vi "BioFeedback4(DAQ+ModularDesign).vi"() -> ()   [LabVIEW 2016]
uses:
  <vilib>/Analysis/5stat.llb/RMS (DBL).vi
  <vilib>/Analysis/NI_AALPro.lvlib
panel:
  out "initialized array size 2":dbl
  in  "Frames Per Second 2":dbl
  in  "Sample rate (Hz) 2":dbl=22050.0 caption="Sample rate (Hz)"
  out "Thermometer Elapsed Frames 2":i32
  out "(INTERNAL) Buffer Index 2":i32
  out "Moving Average num samples 2":i32
  out "AggregateSignalData 2":waveform(dbl)[](array[waveform])
  in  "Moving Average Length (s) 2":dbl
  out "rectified 4":waveform(dbl)[](graph)
  out "Data Levels 2":dbl(slide) scale=0.0..0.07
  out "rms data 2":dbl(graph)
  out "rectified 3":waveform(dbl)[](graph)
  out "raw input 2":waveform(dbl)(graph)
  out "aggregate signal 2":waveform(dbl)[](graph)
  out "initialized array size":dbl
  out "rectified 2":waveform(dbl)[](graph)
  out "number of resets":dbl
  in  "Frames Per Second":dbl
  in  "Sample rate (Hz)":dbl=22050.0
  out "Thermometer Elapsed Frames":i32
  out "(INTERNAL) Buffer Index":i32
  out "Moving Average num samples":i32
  out "AggregateSignalData":waveform(dbl)[](array[waveform])
  in  "Moving Average Length (s)":dbl
  out "rectified":waveform(dbl)[](graph)
  out "Data Levels":dbl(slide) scale=0.0..0.07
  out "rms data":dbl(graph)
  out "raw input":waveform(dbl)(graph)
  out "aggregate signal":waveform(dbl)[](graph)
  in  "Trial":dbl
  in  "Start":bool
  in  "Stop Recording":bool
  # "Biofeedback"
  # "Internal"
  # "Settings"
  # "Filter Settings"
  # "Bandpass Filter"
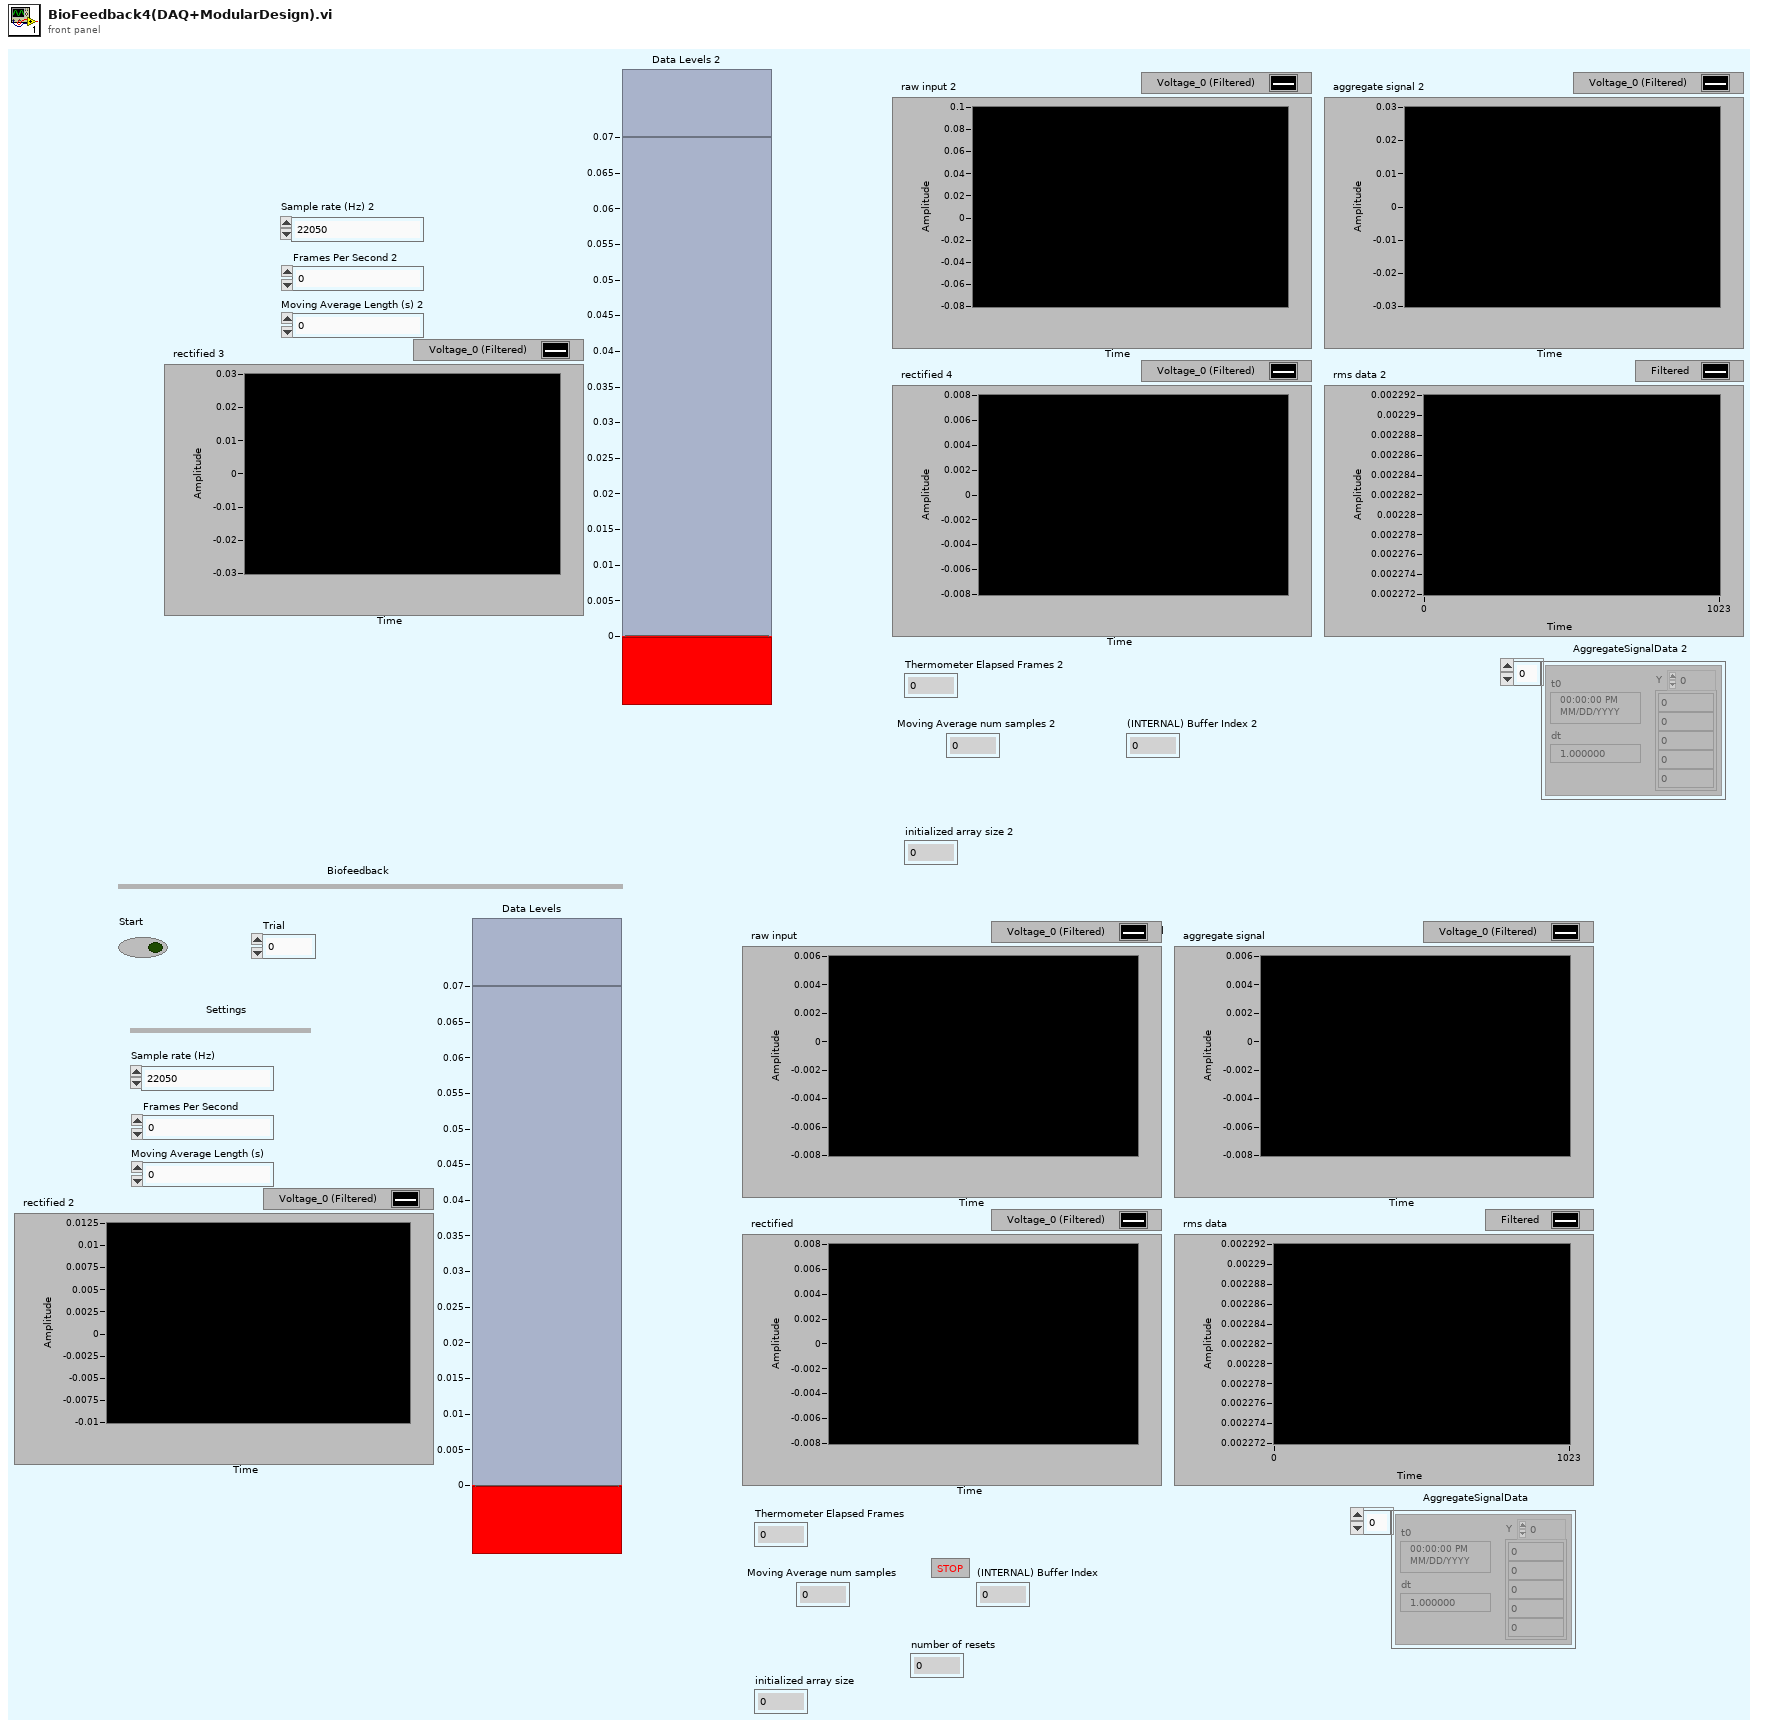
[diagram p1: front panel]
types:
  T1 = typedef "WaveformArrayControl.ctl" = waveform(dbl)[]
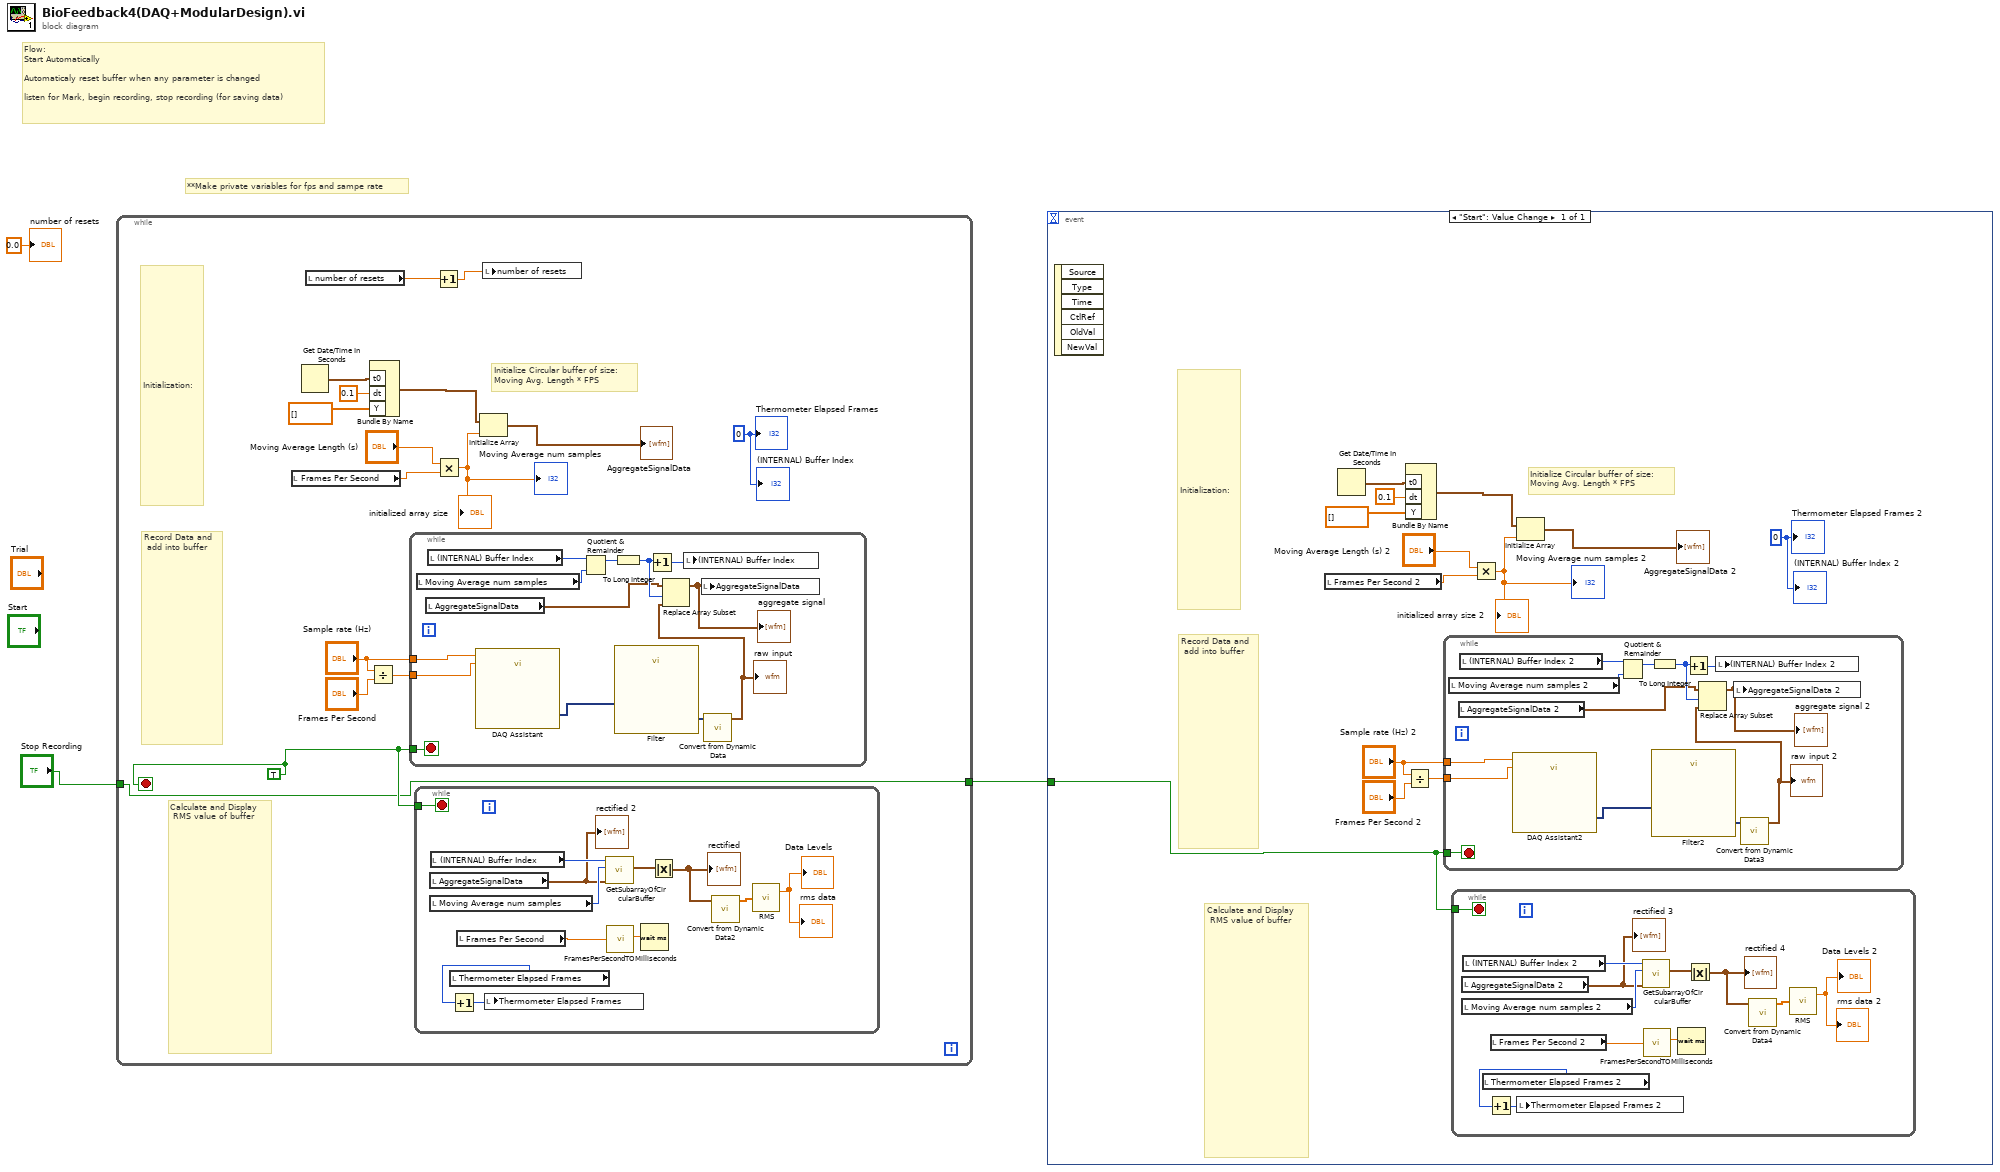
[diagram p0: block diagram]
diagram:
  # "**Make private variables for fps and sampe rate"
  # "Flow:\nStart Automatically\n\nAutomaticaly reset buffer when any parameter is changed\n\nlisten for Mark, begin recording, stop recording (for saving data)"
  n1 = while {
    tunnel: "Stop Recording" -> [w4]
    tunnel: [w4] -> w1
    stop <- w5 stop-if-true
    w5 = TRUE
    w17 = 0 ("Thermometer Elapsed Frames")
    # "Initialization:"
    # "Initialize Circular buffer of size:\nMoving Avg. Length * FPS"
    # "Record Data and\n add into buffer"
    # "Calculate and Display\n RMS value of buffer"
    n2 = local read "Frames Per Second"() -> (w19:dbl)
    n3 = Get Date/Time In Seconds() -> (seconds since 1Jan1904=w12:timestamp)
    n4 = local read "number of resets"() -> (w8:dbl)
    n5 = Bundle By Name("t0"=w12, "dt"=0.1, "Y"=dbl[] []) -> (w9:waveform(dbl))  [unwired: 1 in]
    n6 = Divide(x="Sample rate (Hz)", y="Frames Per Second") -> (x/y=w14:dbl)
    n7 = while {
      tunnel: "Sample rate (Hz)" -> [w41]
      tunnel: w14 -> [w40]
      tunnel: w5 -> [w32]
      stop <- w32 stop-if-true
      n8 = local read "Moving Average num samples"() -> (w44:i32)
      n9 = local read "AggregateSignalData"() -> (w35:waveform(dbl)[])
      n10 = local read "(INTERNAL) Buffer Index"() -> (w43:i32)
      n11 = call "DAQ Assistant"("rate"=w41, "number of samples"=w40) -> ("data"=w38:dynamicdata)  [unwired: 15 in, 2 out]
      n12 = Quotient & Remainder(x=w43, y=w44) -> (x-y*floor(x/y)=w39:i32)  [unwired: 1 out]
      n13 = To Long Integer(number=w39) -> (32bit integer=w36:i32)
      n14 = call "Filter"("Signal"=w38) -> ("Filtered Signal"=w37:dynamicdata)  [unwired: 9 in, 1 out]
      n15 = Increment(x=w36) -> (x+1=w42:i32)
      n16 = local write "(INTERNAL) Buffer Index"(w42) -> ()
      n17 = call "Convert from Dynamic Data"("Dynamic Data Type"=w37) -> ("Waveform"=w34:waveform(dbl))  [unwired: 3 in]
      "raw input" <- w34
      n18 = Replace Array Subset(array=w35, new element=w34, index=w36) -> (w33:waveform(dbl)[])
      "aggregate signal" <- w33
      n19 = local write "AggregateSignalData"(w33) -> ()
    }
    n20 = while {
      tunnel: w5 -> [w20]
      stop <- w20 stop-if-true
      n21 = local read "AggregateSignalData"() -> (w21:waveform(dbl)[])
      "rectified 2" <- w21
      n22 = local read "Moving Average num samples"() -> (w26:i32)
      n23 = local read "(INTERNAL) Buffer Index"() -> (w25:i32)
      n24 = local read "Thermometer Elapsed Frames"() -> (w30:i32)
      n25 = Increment(x=w30) -> (x+1=w29:i32)
      n26 = local read "Frames Per Second"() -> (w28:dbl)
      n27 = local write "Thermometer Elapsed Frames"(w29) -> ()
      n28 = call "GetSubarrayOfCircularBuffer.vi"("initialized array"=w21, "subset size"=w26, "start index"=w25) -> ("initialized array 2"=w24:T1)  [unwired: 8 in]
      n29 = call "FramesPerSecondTOMilliseconds.vi"("Thermometer\nFps"=w28) -> ("x*y"=w31:dbl)  [unwired: 10 in]
      n30 = Wait (ms)(milliseconds to wait=w31) -> ()  [unwired: 1 out]
      n31 = Absolute Value(x=w24) -> (abs(x)=w23:T1)
      "rectified" <- w23
      n32 = call "Convert from Dynamic Data2"("Dynamic Data Type"=w23) -> ("Array"=w22:dbl[])  [unwired: 3 in]
      n33 = call-poly <vilib>:"RMS.vi"("X"=w22) -> ("rms value"=→"Data Levels" →"rms data":dbl)  [unwired: 1 out]
    }
    n34 = Increment(x=w8) -> (x+1=w7:dbl)
    n35 = Multiply(x="Moving Average Length (s)", y=w19) -> (x*y=w6:dbl)
    "Moving Average num samples" <- w6
    "initialized array size" <- w6
    n36 = Initialize Array(w9, w6) -> (→"AggregateSignalData":waveform(dbl)[])
    n37 = local write "number of resets"(w7) -> ()
    "(INTERNAL) Buffer Index" <- w17
    "Thermometer Elapsed Frames" <- w17
  }
  n38 = event shown="[0] \"Start\": Value Change" {
    selector: _ -> [_]
    dyn-events: _ -> [_]
    timeout: _ -> [_]
    tunnel: w1 -> [w45]
    event "Start": Value Change {
      w55 = 0 ("Thermometer Elapsed Frames")
      # "Initialization:"
      # "Initialize Circular buffer of size:\nMoving Avg. Length * FPS"
      # "Record Data and\n add into buffer"
      # "Calculate and Display\n RMS value of buffer"
      n39 = event-data() -> ()  [unwired: 1 in, 6 out]
      n40 = local read "Frames Per Second 2"() -> (w57:dbl)
      n41 = Get Date/Time In Seconds() -> (seconds since 1Jan1904=w50:timestamp)
      n42 = Bundle By Name("t0"=w50, "dt"=0.1, "Y"=dbl[] []) -> (w47:waveform(dbl))  [unwired: 1 in]
      n43 = Divide(x="Sample rate (Hz) 2", y="Frames Per Second 2") -> (x/y=w52:dbl)
      n44 = while {
        tunnel: "Sample rate (Hz) 2" -> [w79]
        tunnel: w52 -> [w78]
        tunnel: w45 -> [w70]
        stop <- w70 stop-if-true
        n45 = local read "Moving Average num samples 2"() -> (w82:i32)
        n46 = local read "AggregateSignalData 2"() -> (w73:waveform(dbl)[])
        n47 = local read "(INTERNAL) Buffer Index 2"() -> (w81:i32)
        n48 = call "DAQ Assistant2"("rate"=w79, "number of samples"=w78) -> ("data"=w76:dynamicdata)  [unwired: 15 in, 2 out]
        n49 = Quotient & Remainder(x=w81, y=w82) -> (x-y*floor(x/y)=w77:i32)  [unwired: 1 out]
        n50 = To Long Integer(number=w77) -> (32bit integer=w74:i32)
        n51 = call "Filter2"("Signal"=w76) -> ("Filtered Signal"=w75:dynamicdata)  [unwired: 9 in, 1 out]
        n52 = Increment(x=w74) -> (x+1=w80:i32)
        n53 = local write "(INTERNAL) Buffer Index 2"(w80) -> ()
        n54 = call "Convert from Dynamic Data3"("Dynamic Data Type"=w75) -> ("Waveform"=w72:waveform(dbl))  [unwired: 3 in]
        "raw input 2" <- w72
        n55 = Replace Array Subset(array=w73, new element=w72, index=w74) -> (w71:waveform(dbl)[])
        "aggregate signal 2" <- w71
        n56 = local write "AggregateSignalData 2"(w71) -> ()
      }
      n57 = while {
        tunnel: w45 -> [w58]
        stop <- w58 stop-if-true
        n58 = local read "AggregateSignalData 2"() -> (w59:waveform(dbl)[])
        "rectified 3" <- w59
        n59 = local read "Moving Average num samples 2"() -> (w64:i32)
        n60 = local read "(INTERNAL) Buffer Index 2"() -> (w63:i32)
        n61 = local read "Thermometer Elapsed Frames 2"() -> (w68:i32)
        n62 = Increment(x=w68) -> (x+1=w67:i32)
        n63 = local read "Frames Per Second 2"() -> (w66:dbl)
        n64 = local write "Thermometer Elapsed Frames 2"(w67) -> ()
        n65 = call "GetSubarrayOfCircularBuffer.vi"("initialized array"=w59, "subset size"=w64, "start index"=w63) -> ("initialized array 2"=w62:T1)  [unwired: 8 in]
        n66 = call "FramesPerSecondTOMilliseconds.vi"("Thermometer\nFps"=w66) -> ("x*y"=w69:dbl)  [unwired: 10 in]
        n67 = Wait (ms)(milliseconds to wait=w69) -> ()  [unwired: 1 out]
        n68 = Absolute Value(x=w62) -> (abs(x)=w61:T1)
        "rectified 4" <- w61
        n69 = call "Convert from Dynamic Data4"("Dynamic Data Type"=w61) -> ("Array"=w60:dbl[])  [unwired: 3 in]
        n70 = call-poly <vilib>:"RMS.vi"("X"=w60) -> ("rms value"=→"Data Levels 2" →"rms data 2":dbl)  [unwired: 1 out]
      }
      n71 = Multiply(x="Moving Average Length (s) 2", y=w57) -> (x*y=w46:dbl)
      "Moving Average num samples 2" <- w46
      "initialized array size 2" <- w46
      n72 = Initialize Array(w47, w46) -> (→"AggregateSignalData 2":waveform(dbl)[])
      "(INTERNAL) Buffer Index 2" <- w55
      "Thermometer Elapsed Frames 2" <- w55
    }
  }
  "number of resets" <- 0.0 ("number of resets")
